vi "Leaderboard test 4.vi"() -> ()   [LabVIEW 2020, in "Visualisation.lvclass"]
uses:
  Visualisation.lvclass
  Application/Globals.vi
  Data Manager/Data Manager.lvclass
  Application/Application.lvlib
panel:
  out "Walk":T1(array[cluster]) {"Distance 2" scale=0.0..59.162}
  out "Leaderboard":T2(array[cluster]) {"Distance" scale=0.0..117.46605}
  out "Ride":T3(array[cluster]) {"Distance 4" scale=0.0..53.09895}
  out "Run":T4(array[cluster]) {"Distance 3" scale=0.0..63.102}
  out "B Total":dbl format="%0.1f km"
  out "A Total":dbl format="%0.1f km"
  # "Total Distance Leaderboard"
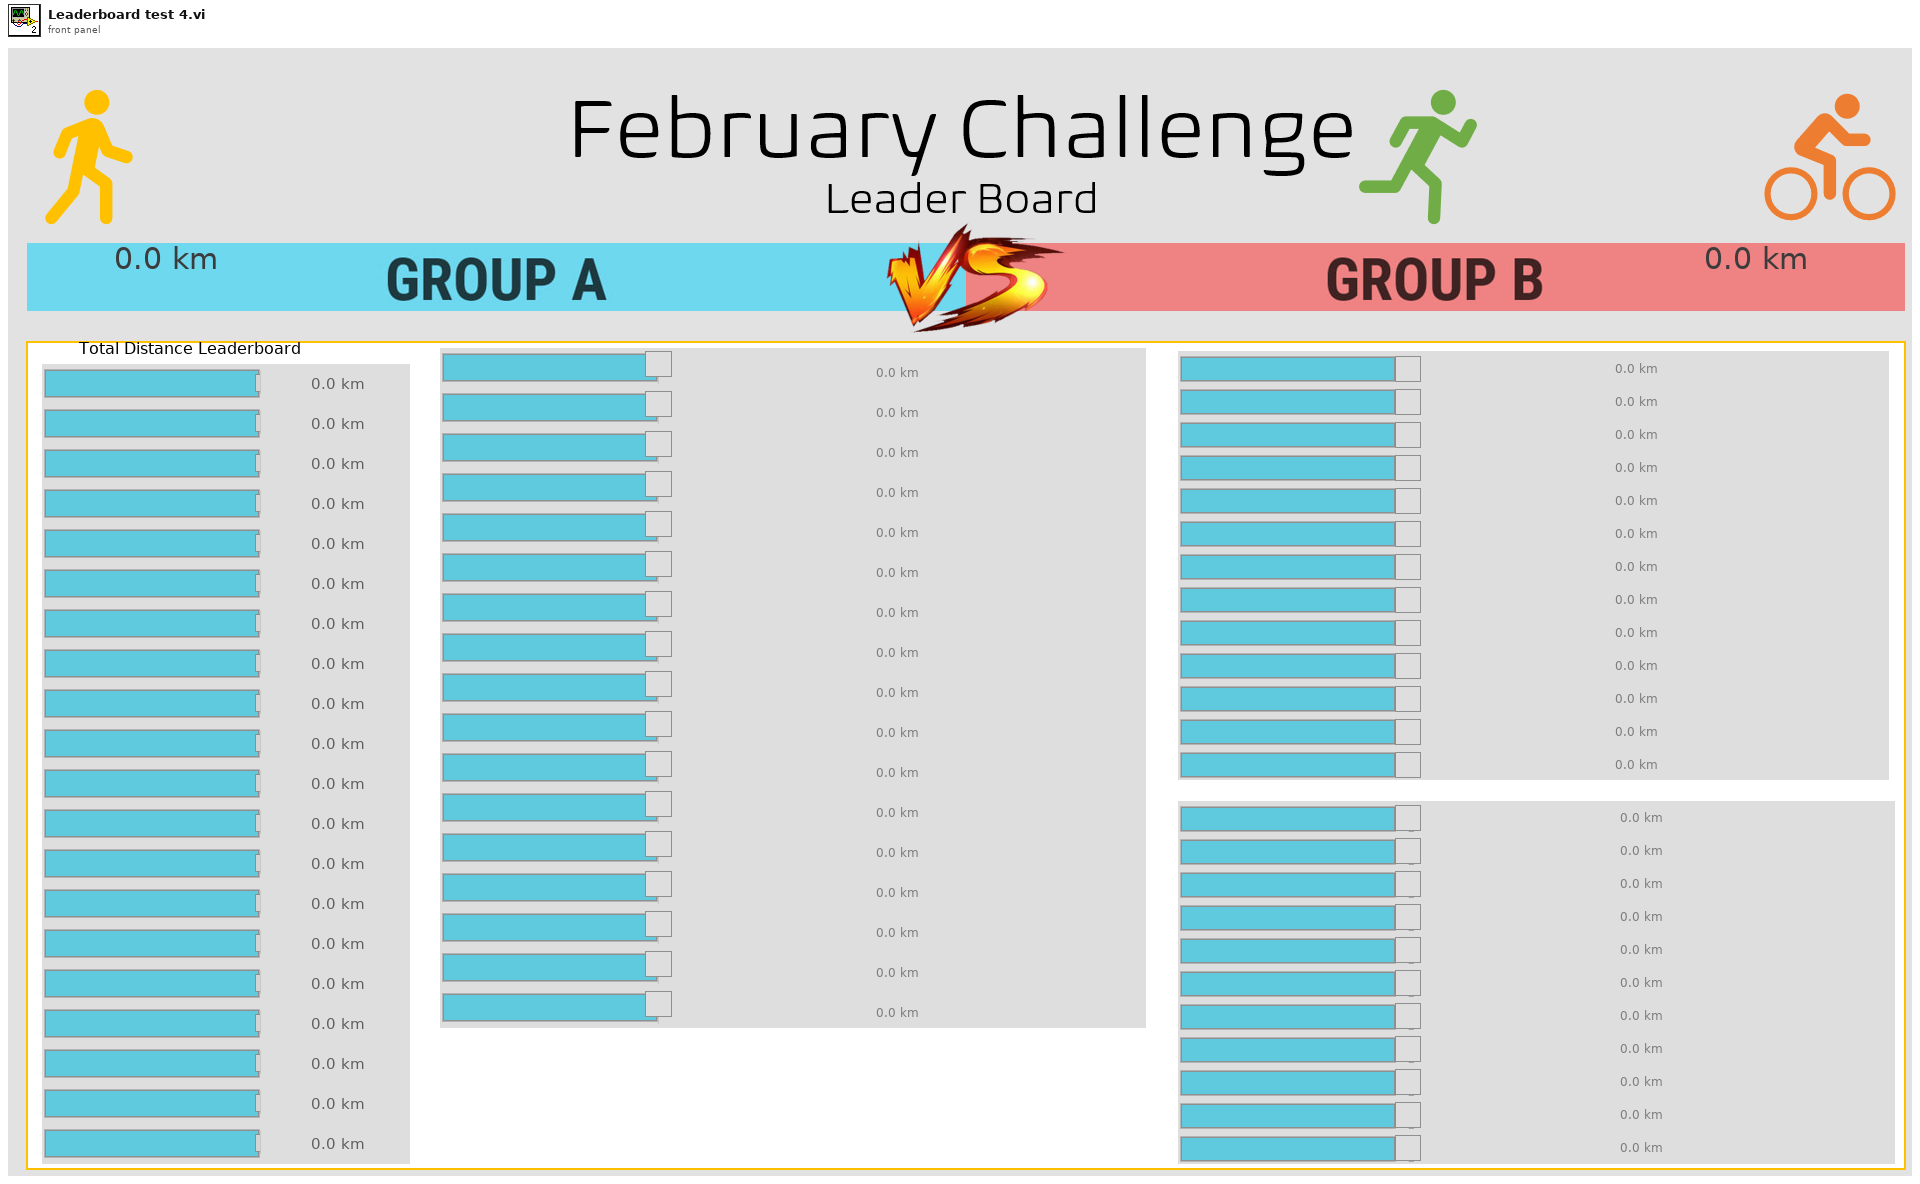
[diagram p1: front panel]
types:
  T1 = cluster{"Athlete":string, "Team":u32, "Distance 2":dbl}[]
  T2 = cluster{"Athlete":string, "Distance":dbl, "Team":u32}[]
  T3 = cluster{"Athlete":string, "Team":u32, "Distance 4":dbl}[]
  T4 = cluster{"Athlete":string, "Team":u32, "Distance 3":dbl}[]
  T5 = cluster{"Athlete":string, "Team":u32, "Distance 2":dbl}
  T6 = cluster{"Athlete":string, "Distance":dbl, "Team":u32, "Distance 2":cluster{"Numeric":dbl, "Numeric":dbl, "Numeric":dbl}}
  T7 = cluster{"Athlete":string, "Distance":dbl, "Team":u32}
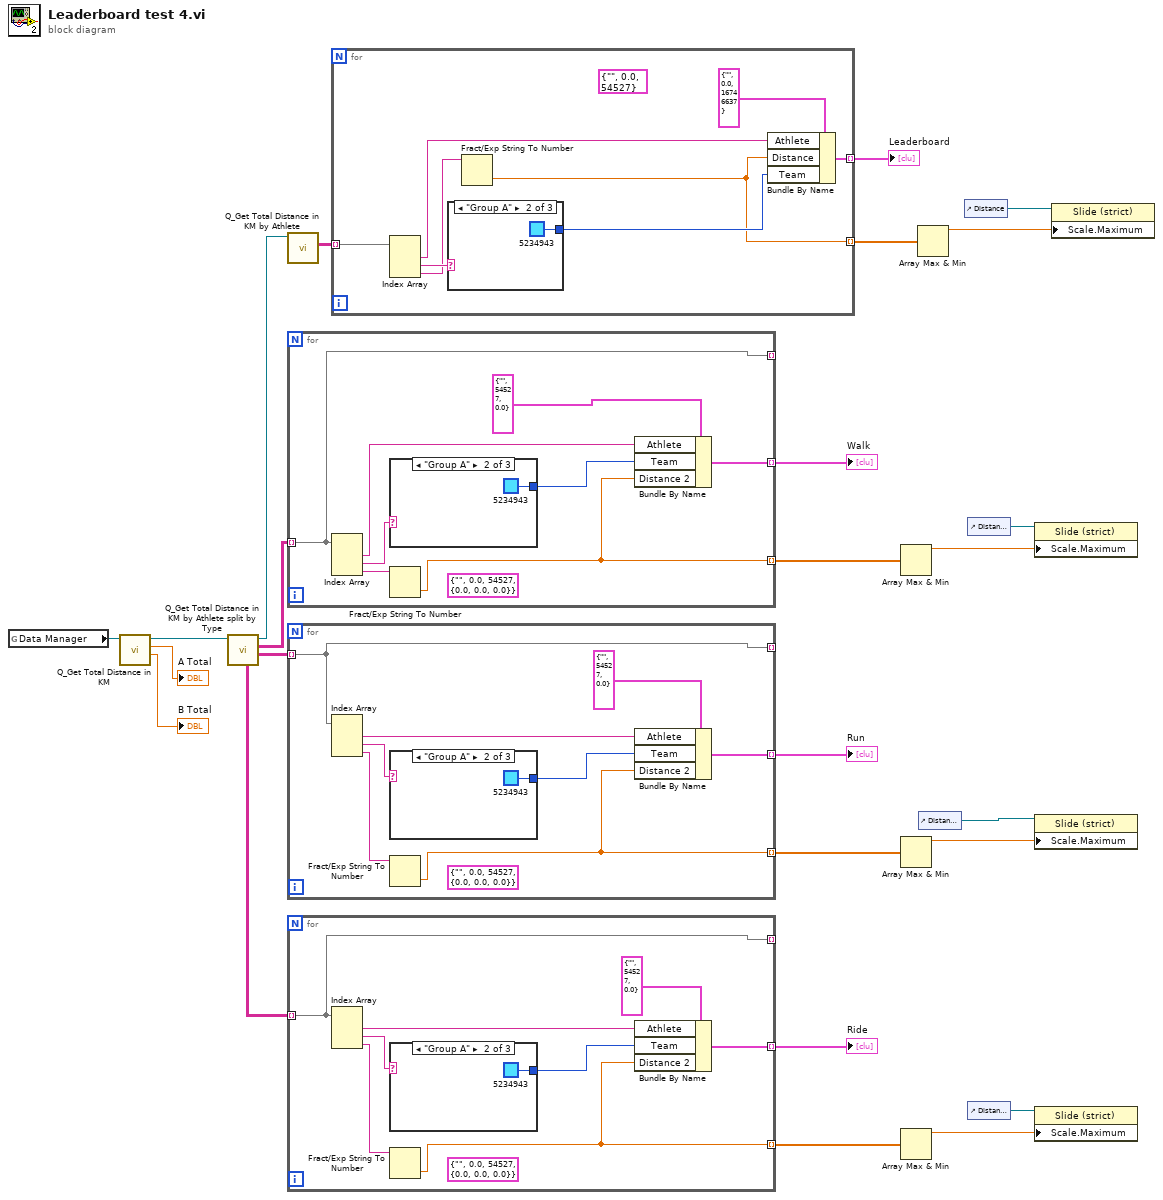
[diagram p0: block diagram]
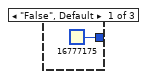
[diagram p2: hidden frame]
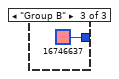
[diagram p3: hidden frame]
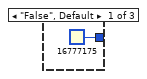
[diagram p4: hidden frame]
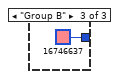
[diagram p5: hidden frame]
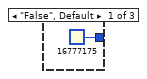
[diagram p6: hidden frame]
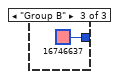
[diagram p7: hidden frame]
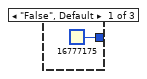
[diagram p8: hidden frame]
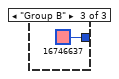
[diagram p9: hidden frame]
diagram:
  n1 = global read "Globals.vi" "Data Manager"() -> (w25:refnum<class "Data Manager.lvclass">)
  n2 = call-dynamic "Q_Get Total Distance in KM.vi"("Data Manager in"=w25) -> ("Group B"=→"B Total":dbl, "Group A"=→"A Total":dbl, "Data Manager out"=w20:refnum<class "Data Manager.lvclass">)  [unwired: 6 in, 2 out]
  n3 = call-dynamic "Q_Get Total Distance in KM by Athlete split by Type.vi"("Data Manager in"=w20) -> ("Run"=w15:string[][], "Walk"=w19:string[][], "Data Manager out"=w8:refnum<class "Data Manager.lvclass">, "Ride"=w12:string[][])  [unwired: 6 in, 1 out]
  n4 = call-dynamic "Q_Get Total Distance in KM by Athlete.vi"("Data Manager in"=w8) -> ("Result Set"=w7:string[][])  [unwired: 8 in, 2 out]
  n5 = for {
    tunnel: [w28] -> _ mode=indexing
    tunnel: [w33] -> w1 mode=indexing
    tunnel: w19 -> [w28] mode=indexing
    tunnel: [w27] -> w16 mode=indexing
    (unwired) T6 {"Athlete"="", "Distance"=0.0, "Team"=54527, "Distance 2"={"Numeric"=0.0, "Numeric"=0.0, "Numeric"=0.0}} ("Leaderboard")
    n6 = Index Array(array=w28) -> (element #1=w29:string, element #2=w31:string, element #3=w30:string)  [unwired: 3 in]
    n7 = case shown="\"Group A\"" w31 {
      tunnel: [u32 16777175 ("Color Box") u32 5234943 ("Color Box") u32 16746637 ("Color Box")] -> w32
      frame "False", Default {
      }
      frame "Group A" {
      }
      frame "Group B" {
      }
    }
    n8 = Fract/Exp String To Number(string=w30) -> (number=w27:dbl)  [unwired: 3 in, 1 out]
    n9 = Bundle By Name(cluster=T5 {"Athlete"="", "Team"=54527, "Distance 2"=0.0} ("Leaderboard"), "Athlete"=w29, "Team"=w32, "Distance 2"=w27) -> (w33:T5)
  }
  "Walk" <- w1
  n10 = for {
    tunnel: w15 -> [w39] mode=indexing
    tunnel: [w44] -> w13 mode=indexing
    tunnel: [w39] -> _ mode=indexing
    tunnel: [w38] -> w14 mode=indexing
    (unwired) T6 {"Athlete"="", "Distance"=0.0, "Team"=54527, "Distance 2"={"Numeric"=0.0, "Numeric"=0.0, "Numeric"=0.0}} ("Leaderboard")
    n11 = Index Array(array=w39) -> (element #1=w40:string, element #2=w42:string, element #3=w41:string)  [unwired: 3 in]
    n12 = case shown="\"Group A\"" w42 {
      tunnel: [u32 16777175 ("Color Box") u32 5234943 ("Color Box") u32 16746637 ("Color Box")] -> w43
      frame "False", Default {
      }
      frame "Group A" {
      }
      frame "Group B" {
      }
    }
    n13 = Fract/Exp String To Number(string=w41) -> (number=w38:dbl)  [unwired: 3 in, 1 out]
    n14 = Bundle By Name(cluster=T5 {"Athlete"="", "Team"=54527, "Distance 2"=0.0} ("Leaderboard"), "Athlete"=w40, "Team"=w43, "Distance 2"=w38) -> (w44:T5)
  }
  "Run" <- w13
  n15 = for {
    tunnel: w12 -> [w50] mode=indexing
    tunnel: [w55] -> w10 mode=indexing
    tunnel: [w50] -> _ mode=indexing
    tunnel: [w49] -> w11 mode=indexing
    (unwired) T6 {"Athlete"="", "Distance"=0.0, "Team"=54527, "Distance 2"={"Numeric"=0.0, "Numeric"=0.0, "Numeric"=0.0}} ("Leaderboard")
    n16 = Index Array(array=w50) -> (element #1=w51:string, element #2=w53:string, element #3=w52:string)  [unwired: 3 in]
    n17 = case shown="\"Group A\"" w53 {
      tunnel: [u32 16777175 ("Color Box") u32 5234943 ("Color Box") u32 16746637 ("Color Box")] -> w54
      frame "False", Default {
      }
      frame "Group A" {
      }
      frame "Group B" {
      }
    }
    n18 = Fract/Exp String To Number(string=w52) -> (number=w49:dbl)  [unwired: 3 in, 1 out]
    n19 = Bundle By Name(cluster=T5 {"Athlete"="", "Team"=54527, "Distance 2"=0.0} ("Leaderboard"), "Athlete"=w51, "Team"=w54, "Distance 2"=w49) -> (w55:T5)
  }
  "Ride" <- w10
  n20 = for {
    tunnel: w7 -> [w65] mode=indexing
    tunnel: [w66] -> w6 mode=indexing
    tunnel: [w59] -> w4 mode=indexing
    (unwired) T7 {"Athlete"="", "Distance"=0.0, "Team"=54527} ("Leaderboard")
    n21 = Index Array(array=w65) -> (element #1=w61:string, element #2=w63:string, element #3=w62:string)  [unwired: 3 in]
    n22 = case shown="\"Group A\"" w63 {
      tunnel: [u32 16777175 ("Color Box") u32 5234943 ("Color Box") u32 16746637 ("Color Box")] -> w64
      frame "False", Default {
      }
      frame "Group A" {
      }
      frame "Group B" {
      }
    }
    n23 = Fract/Exp String To Number(string=w62) -> (number=w59:dbl)  [unwired: 3 in, 1 out]
    n24 = Bundle By Name(cluster=T7 {"Athlete"="", "Distance"=0.0, "Team"=16746637} ("Leaderboard"), "Athlete"=w61, "Distance"=w59, "Team"=w64) -> (w66:T7)
  }
  "Leaderboard" <- w6
  n25 = Array Max & Min(array=w16) -> (max value=w17:dbl)  [unwired: 3 out]
  n26 = Array Max & Min(array=w14) -> (max value=w22:dbl)  [unwired: 3 out]
  n27 = Array Max & Min(array=w11) -> (max value=w21:dbl)  [unwired: 3 out]
  n28 = Array Max & Min(array=w4) -> (max value=w5:dbl)  [unwired: 3 out]
  n29 = control-ref of="Distance 3"() -> (w2:refnum<vi>)
  n30 = control-ref of="Distance"() -> (w3:refnum<vi>)
  n31 = control-ref of="Distance 2"() -> (w18:refnum<vi>)
  n32 = control-ref of="Distance 4"() -> (w9:refnum<vi>)
  n33 = property on="Property Node" class="Slide (strict)"(reference=w18, "Scale.Maximum"=w17) -> ()  [unwired: 1 in, 2 out]
  n34 = property on="Property Node" class="Slide (strict)"(reference=w2, "Scale.Maximum"=w22) -> ()  [unwired: 1 in, 2 out]
  n35 = property on="Property Node" class="Slide (strict)"(reference=w9, "Scale.Maximum"=w21) -> ()  [unwired: 1 in, 2 out]
  n36 = property on="Property Node" class="Slide (strict)"(reference=w3, "Scale.Maximum"=w5) -> ()  [unwired: 1 in, 2 out]
